vi "LV_MAIN.vi"() -> ()   [LabVIEW 2010]
uses:
  idd.vi
  global1.vi
  <vilib>/Utility/file.llb/Read From Spreadsheet File (DBL).vi
  <vilib>/Utility/file.llb/Write To Spreadsheet File (DBL).vi
panel:
  out "实际位移（AD）":dbl=150.0
  out "输出电压报警":bool
  in  "开始":bool
  in  "停止":bool
  in  "暂停波形":bool
  in  "读取波形":bool
  in  "保存波形":bool
  out "波形图表":dbl(graph)
  in  "table":enum32{"实时值", "参数设置"}(tab)
  in  "周期(ms)":u32=50
  in  "执行次数":u32=100
  in  "PID参数":cluster{"微分系数":dbl, "积分系数":dbl, "比例系数":dbl}
  in  "方式":enum32{"阶跃", "正弦", "方波"}(tab)
  in  "目标位移（给定值）":dbl=150.0
  in  "正弦参数":cluster{"幅值(mm)":dbl, "中心(mm)":dbl}={"幅值(mm)"=50.0, "中心(mm)"=100.0}
  in  "方波参数":cluster{"目标位移1":dbl, "目标位移2":dbl, "占空比":dbl}={"目标位移1"=150.0, "目标位移2"=100.0, "占空比"=50.0}
  in  "采样点数":i32=10
  in  "AD通道选择":i32
  in  "DA通道选择":i32=1 min=0 max=1
  in  "输出电压上限(V)":dbl
  in  "输出电压下限(V)":dbl
  # "PID参数设置"
  # "板卡AC_6011参数设置"
  # "滤波参数"
  # "输出电压保护参数"
  # "给定值"
  # "位移"
  # "PID控制算法"
  # "D/A"
  # "减速器"
  # "伺服电源"
  # "直流伺服电机"
  # "滚珠丝杆"
  # "负载"
  # "位移传感器"
  # "A/D"
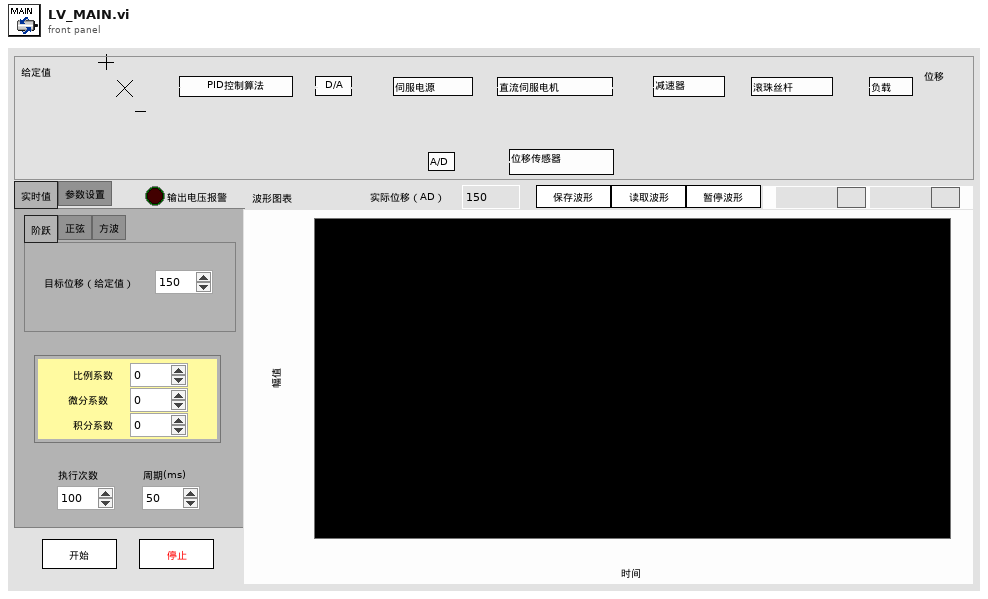
[diagram p1: front panel]
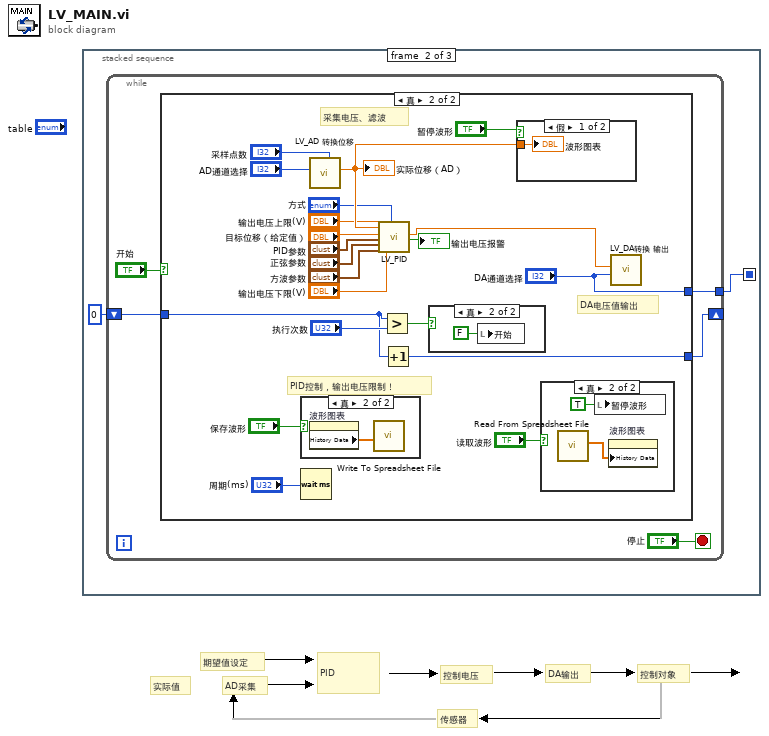
[diagram p0: block diagram]
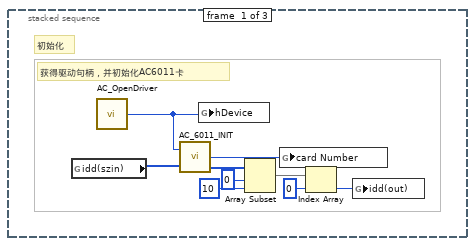
[diagram p2: hidden frame]
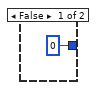
[diagram p3: hidden frame]
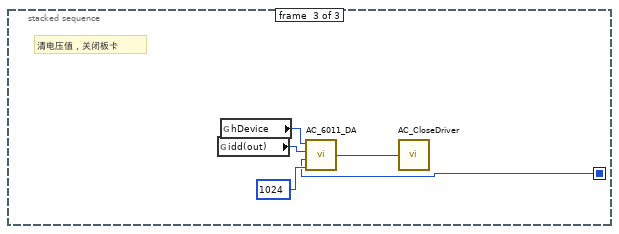
[diagram p8: hidden frame]
diagram:
  # "传感器"
  # "控制对象"
  # "DA输出"
  # "控制电压"
  # "AD采集"
  # "PID"
  # "实际值"
  # "期望值设定"
  n1 = stacked-sequence {
    seq-local: [_ w11 _] -> [_ _ w44]
    frame #0 {
      # "获得驱动句柄，并初始化AC6011卡"
      # "初始化"
      n2 = global read "idd.vi" "idd(szin)"() -> (w6:u32[])
      n3 = call "AC_OpenDriver.vi"() -> ("hDevice"=w5:u32)  [unwired: 1 in]
      n4 = call "AC_6011_INIT.vi"("hDevice(in)"=w5, "idd(szin)"=w6) -> ("Cardc"=w4:i32, "idd(szout)"=w7:u32[])  [unwired: 1 out]
      n5 = global write "idd.vi" "hDevice"(w5) -> ()
      n6 = Array Subset(array=w7, index=0, length=10) -> (w2:u32[])
      n7 = global write "global1.vi" "card Number"(w4) -> ()
      n8 = Index Array(array=w2, index=0 ("索引")) -> (element=w3:u32)
      n9 = global write "idd.vi" "idd(out)"(w3) -> ()
    }
    frame #1 {
      n10 = while {
        tunnel: [w15] -> w11
        shift-right: [w12] -> _
        shift-left: u32 0 -> [w13]
        stop <- "停止" stop-if-true
        n11 = case shown="真" "开始" {
          tunnel: [_ "DA通道选择"] -> w15
          tunnel: w13 -> [_ w18]
          tunnel: [u32 0 w20] -> w12
          frame False {
          }
          frame True {
            # "采集电压、滤波"
            # "DA电压值输出"
            # "PID控制，输出电压限制！"
            n12 = case shown="真" "保存波形" {
              frame False {
              }
              frame True {
                n13 = property on="波形图表" class="WFChart (严格)"() -> ("History Data"=w43:dbl[])  [unwired: 2 in, 2 out]
                n14 = call-poly <vilib>:"Write To Spreadsheet File.vi"("1D data"=w43) -> ()  [unwired: 7 in, 1 out]
              }
            }
            n15 = Wait (ms)(milliseconds to wait="周期(ms)") -> ()  [unwired: 1 out]
            n16 = call "LV_AD 转换位移.vi"("采样次数"="采样点数", "AD通道"="AD通道选择") -> ("实际位移"=w30:dbl)  [unwired: 9 in]
            "实际位移（AD）" <- w30
            n17 = call "LV_PID.vi"("实际位移"=w30, "目标位移"="目标位移（给定值）", "PID参数"="PID参数", "正弦参数"="正弦参数", "方波参数"="方波参数", "输出电压上限"="输出电压上限(V)", "输出电压下限"="输出电压下限(V)", "方式"="方式") -> ("输出电压"=w35:dbl, "输出电压极限报警"=→"输出电压报警":bool)  [unwired: 10 in]
            n18 = Greater?(x=w18, y="执行次数") -> (0:w19:bool)
            n19 = Increment(x=w18) -> (x+1=w20:u32)
            n20 = case shown="真" w19 {
              frame False {
              }
              frame True {
                n21 = local write "开始"(FALSE ("开始")) -> ()
              }
            }
            n22 = case shown="假" "暂停波形" {
              tunnel: w30 -> [w40 _]
              frame False {
                "波形图表" <- w40
              }
              frame True {
              }
            }
            n23 = case shown="真" "读取波形" {
              frame False {
              }
              frame True {
                n24 = call-poly <vilib>:"Read From Spreadsheet File.vi"() -> ("first row"=w42:dbl[])  [unwired: 7 in, 4 out]
                n25 = local write "暂停波形"(TRUE ("暂停波形")) -> ()
                n26 = property on="波形图表" class="WFChart (严格)"("History Data"=w42) -> ()  [unwired: 2 in, 2 out]
              }
            }
            n27 = call "LV_DA转换 输出.vi"("DA通道"="DA通道选择", "输入电压"=w35) -> ()  [unwired: 10 in]
          }
        }
      }
    }
    frame #2 {
      # "清电压值，关闭板卡"
      n28 = global read "idd.vi" "idd(out)"() -> (w47:u32)
      n29 = global read "idd.vi" "hDevice"() -> (w48:u32)
      n30 = call "AC_6011_DA.vi"("DAData"=1024, "DAch"=w44, "idd(out)"=w47, "hDevice"=w48) -> ("hDevice(out)"=w46:i32)
      n31 = call "AC_CloseDriver.vi"("hDevice(in)"=w46) -> ()  [unwired: 1 out]
    }
  }
